vi "SimplePIDexample.vi"() -> ()   [LabVIEW 2020]
uses:
  <vilib>/Platform/TimedLoop/XDataNode/timing_clust.ctl
  <vilib>/Platform/TimedLoop/XDataNode/nitl_modes.ctl
  <vilib>/Platform/TimedLoop/XDataNode/wakeup.ctl
  <vilib>/addons/control/pid/pid.llb/PID (DBL).vi
  <vilib>/platform/TimedLoop/XDataNode/XDataNode.xnode
  <vilib>/Platform/TimedLoop/XDataNode/XDNodeRunTimeDep.lvlib
  <vilib>/addons/control/pid/NI_PID_pid.lvlib
panel:
  in  "stop":bool
  out "Waveform Chart":cluster{dbl, "output":dbl}(graph)
  out "Process variable":dbl
  out "Control output":dbl format="%.2f"
  in  "PID gains":T1={"proportional gain (Kc)"=1.0, "integral time (Ti, min)"=0.01, "derivative time (Td, min)"=0.0} {"derivative time (Td, min)" format="%.3f"; "integral time (Ti, min)" format="%.3f"; "proportional gain (Kc)" format="%.3f"}
  in  "output range":cluster{"output high":dbl, "output low":dbl}={"output high"=10.0, "output low"=0.0} {"output low" format="%.2f"; "output high" format="%.2f"}
  in  "setpoint":dbl=5.0 format="%.2f"
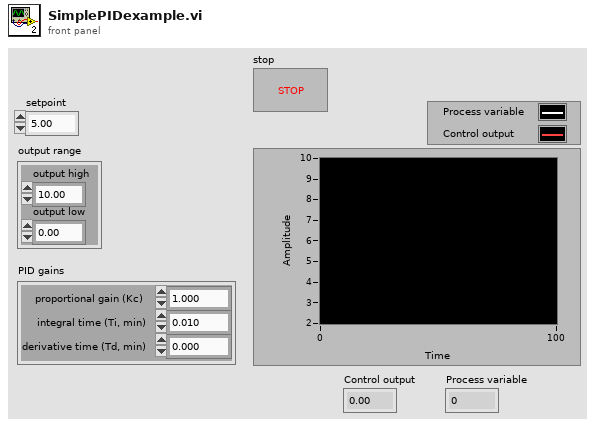
[diagram p1: front panel]
types:
  T1 = cluster{"proportional gain (Kc)":dbl, "integral time (Ti, min)":dbl, "derivative time (Td, min)":dbl}
  T2 = typedef "XDNodeRunTimeDep.lvlib/timing_clust.ctl" = cluster{"Expected End [f-1]":u64, "Actual End [f-1]":u64, "Finished Late? [f-1]":bool, "Expected End [i-1]":u64, "Actual End [i-1]":u64, "Finished Late? [i-1]":bool, "Expected Start [i]":u64, "Actual Start [i]":u64, "Expected Start [f]":u64, "Actual Start [f]":u64, "Source Name":string, "Structure Name":string, "Period":i64, "Deadline":i64, "Offset":i64, "Start":i64, "Priority":i32, "Timeout":i32, "Mode":T3, "Wakeup Reason":T4, "Error":errorcluster, "Source Type":string, "Secondary Source Type":string, "Global End Time":u64, "Global Start Time":u64, "Frame Duration":u64, "Iteration Duration":u64, "Assigned CPU":i32, "I/O Scan Engine Mode":u32}
  T3 = typedef "XDNodeRunTimeDep.lvlib/nitl_modes.ctl" = enum32{"No Change", "Process missed periods, maintain original phase", "Discard missed periods, maintain original phase", "Process missed periods, ignore original phase", "Discard missed periods, ignore original phase"}
  T4 = typedef "XDNodeRunTimeDep.lvlib/wakeup.ctl" = enum32{"Normal", "Aborted", "Asynchronous wakeup", "Timing source error", "Timed loop error", "Timeout"}
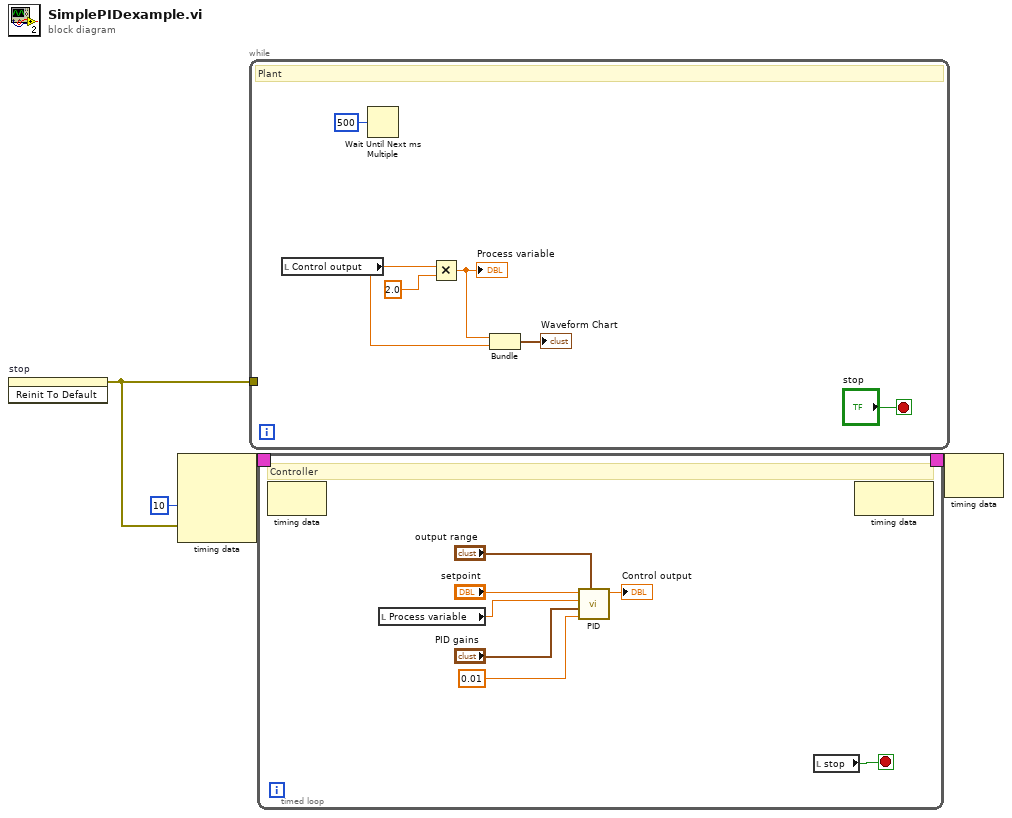
[diagram p0: block diagram]
diagram:
  n1 = invoke on="stop" class="Bool (strict)" method="Reinit To Default"() -> (error out=w1:errorcluster)  [unwired: 3 in, 2 out]
  n2 = node-c288(i64 10 ("Period"), w1) -> (w4:T2)  [unwired: 2 in]
  n3 = while {
    tunnel: w1 -> [_]
    stop <- "stop" stop-if-true
    # "Plant"
    n4 = local read "Control output"() -> (w6:dbl)
    n5 = Wait Until Next ms Multiple(millisecond multiple=u32 500) -> ()  [unwired: 1 out]
    n6 = Multiply(x=w6, y=2.0) -> (x*y=w7:dbl)
    "Process variable" <- w7
    n7 = Bundle(w7, "Control output"=w6) -> (→"Waveform Chart":cluster{dbl, "Control output":dbl})  [unwired: 1 in]
  }
  n8 = timed-loop {
    timing: w4 -> [_]
    timing-out: [_] -> w3
    stop <- w11 stop-if-true
    # "Controller"
    n9 = node-c288() -> ()  [unwired: 1 in, 1 out]
    n10 = local read "Process variable"() -> (w12:dbl)
    n11 = call-poly <vilib>:"PID.vi"("output range"="output range", "dt (s)"=0.01, "PID gains"="PID gains", "process variable"=w12, "setpoint"="setpoint") -> ("output"=→"Control output":dbl)  [unwired: 5 in, 1 out]
    n12 = local read "stop"() -> (w11:bool)
    n13 = node-c288() -> ()  [unwired: 1 in, 1 out]
  }
  n14 = node-c288(w3) -> ()  [unwired: 1 out]
